vi "Outgoing Page.vi"(8 "error in (no error)":errorcluster, 11 "Node Ptr":T1 format="%.0x") -> (0 "error out":errorcluster)   [LabVIEW 2015, in "J1939 Addon System Explorer.lvlib"]
uses:
  J1939 Addon System Explorer.lvlib
  <vilib>/NI Veristand/Custom Device API/Custom Device Item Ref.ctl
  <vilib>/NI VeriStand/Custom Device API/Custom Device API.lvlib
panel:
  in  "SHDocVw.IWebBrowser2":refnum<k7>(container)
types:
  T1 = typedef "Custom Device API.lvlib/Custom Device Item Ref.ctl" = u64
  T2 = typedef "Custom Device API.lvlib/Custom Device Commands.ctl" = enum16{"Default", "Item renamed", "Shutdown", "Dynamic button pressed"}
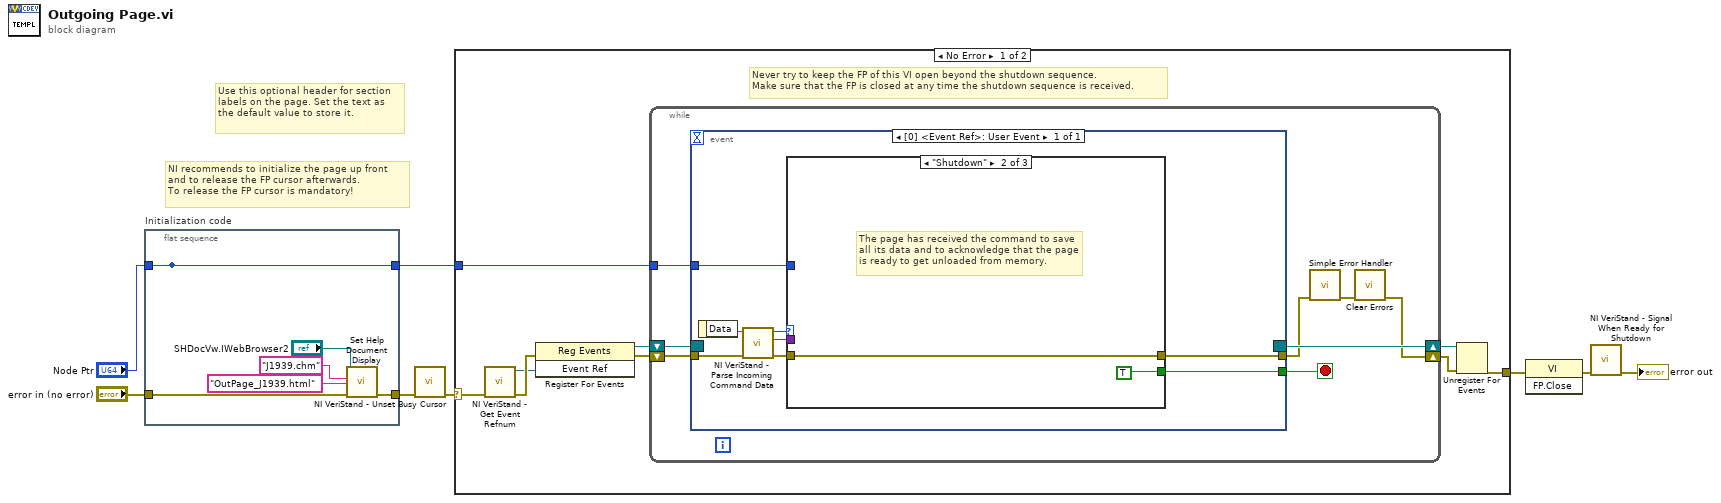
[diagram p0: block diagram]
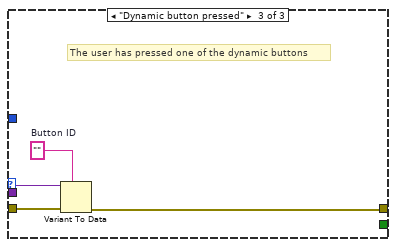
[diagram p3: hidden frame]
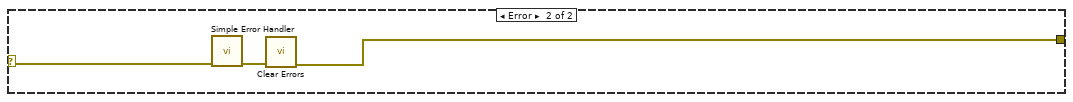
[diagram p4: hidden frame]
diagram:
  # "Use this optional header for section labels on the page. Set the text as the default value to store it."
  # "NI recommends to initialize the page up front\nand to release the FP cursor afterwards.\nTo release the FP cursor is mandatory!"
  n1 = flat-sequence "Initialization code" {
    tunnel: "error in (no error)" -> [w11]
    tunnel: "Node Ptr" -> [w9]
    tunnel: [w10] -> w3
    tunnel: [w9] -> _
    tunnel: [w9] -> w1
    frame #0 {
      n2 = call "Set Help Document Display.vi"("error in (no error)"=w11, "HTML File"="OutPage_J1939.html", "Main CHM File"="J1939.chm", "SHDocVw.IWebBrowser2"="SHDocVw.IWebBrowser2") -> ("error out"=w10:errorcluster)  [unwired: 7 in]
    }
  }
  n3 = call <vilib>:"NI VeriStand - Unset Busy Cursor.vi"("error in (no error)"=w3) -> ("error out"=w5:errorcluster)  [unwired: 10 out]
  n4 = case shown="No Error" w5 {
    selector: w5 -> [w15 w49]
    tunnel: [w20 w47] -> w8
    tunnel: w1 -> [w16 _]
    frame No Error {
      # "Never try to keep the FP of this VI open beyond the shutdown sequence.\nMake sure that the FP is closed at any time the shutdown sequence is received."
      n5 = call <vilib>:"NI VeriStand - Get Event Refnum.vi"("error in (no error)"=w15) -> ("error out"=w23:errorcluster, "Event Ref"=w19:refnum<user-event>)  [unwired: 9 out]
      n6 = register-events(error in=w23, w19) -> (reference out=w17:refnum<event-registration>, error out=w18:errorcluster)  [unwired: 1 in]
      n7 = while {
        tunnel: w16 -> [w27]
        shift-right: [w24] -> w21
        shift-left: w18 -> [w30]
        shift-right: [w31] -> w22
        shift-left: w17 -> [w29]
        stop <- w28 stop-if-true
        n8 = event shown="[0] <Event Ref>: User Event" {
          selector: w29 -> [_]
          dyn-events: [_] -> w31
          timeout: _ -> [_]
          tunnel: w30 -> [w39]
          tunnel: [w35] -> w28
          tunnel: [w34] -> w26
          tunnel: w27 -> [w33]
          event User Event {
            n9 = event-data() -> ("Data"=w38:string)  [unwired: 1 out]
            n10 = call <vilib>:"NI VeriStand - Parse Incoming Command Data.vi"("error in (no error)"=w39, "Incoming data"=w38) -> ("error out"=w37:errorcluster, "Outgoing data"=w32:variant, "Action"=w36:T2)  [unwired: 7 out]
            n11 = case shown="\"Shutdown\"" w36 {
              tunnel: w37 -> [w40 w41 w46]
              tunnel: [_ TRUE _] -> w35
              tunnel: [w40 w41 w43] -> w34
              tunnel: w33 -> [_ _ _]
              tunnel: w32 -> [_ _ w45]
              frame "Default", Default {
              }
              frame "Shutdown" {
                # "The page has received the command to save all its data and to acknowledge that the page is ready to get unloaded from memory."
              }
              frame "Dynamic button pressed" {
                w44 = ""  # Button ID
                # "The user has pressed one of the dynamic buttons"
                n12 = Variant To Data(error in=w46, type=w44, Variant=w45) -> (error out=w43:errorcluster)  [unwired: 1 out]
              }
            }
          }
        }
        n13 = call <vilib>:"Simple Error Handler.vi"("error in (no error)"=w26) -> ("error out"=w25:errorcluster)  [unwired: 1 in, 7 out]
        n14 = call <vilib>:"Clear Errors.vi"("error in (no error)"=w25) -> ("error out"=w24:errorcluster)  [unwired: 1 in, 5 out]
      }
      n15 = Unregister For Events(event registration refnum=w22, error in=w21) -> (error out=w20:errorcluster)
    }
    frame Error {
      n16 = call <vilib>:"Simple Error Handler.vi"("error in (no error)"=w49) -> ("error out"=w48:errorcluster)  [unwired: 1 in, 7 out]
      n17 = call <vilib>:"Clear Errors.vi"("error in (no error)"=w48) -> ("error out"=w47:errorcluster)  [unwired: 1 in, 5 out]
    }
  }
  n18 = invoke class="VI" method="FP.Close"(error in=w8) -> (error out=w7:errorcluster)  [unwired: 2 in, 2 out]
  n19 = call <vilib>:"NI VeriStand - Signal When Ready for Shutdown.vi"("error in (no error)"=w7) -> ("error out"=→"error out":errorcluster)  [unwired: 10 out]
